vi "Global_HW_Status Out.vi"() -> ()   [LabVIEW 2017, in "MechamunDrive.lvlib"]
uses:
  MechamunDrive.lvlib
  Cluster_HW Status.ctl
  TypeDefs/Cluster_SRX Status With Encoder.ctl
panel:
  out "Drive_HW_Status":T1
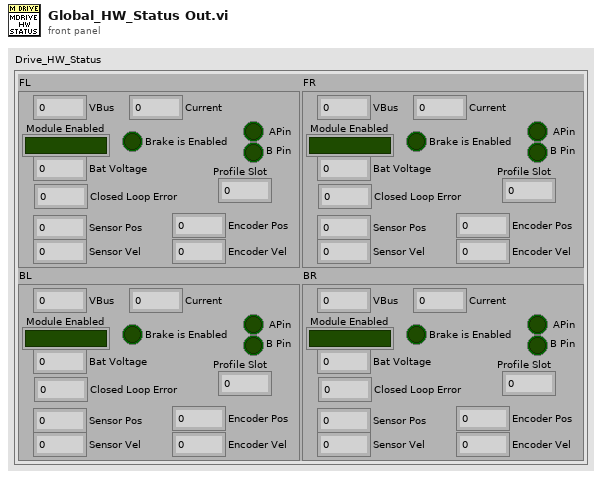
[diagram p1: front panel]
types:
  T1 = typedef "MechamunDrive.lvlib/Cluster_HW Status.ctl" = cluster{"BL":T2, "BR":T2, "FL":T2, "FR":T2}
  T2 = typedef "Cluster_SRX Status With Encoder.ctl" = cluster{"VBus ":dbl, "Module Enabled":bool, "Closed Loop Error":dbl, "Sensor Pos":dbl, "Sensor Vel":dbl, "Current":dbl, "Brake is Enabled":bool, "Encoder Pos":dbl, "Encoder Vel":dbl, " APin":bool, "B Pin":bool, "Bat Voltage":dbl, "Profile Slot":dbl}
diagram:
